vi "Set Project Path.vi"(10 "Top Level Path":path, 11 "Message Enqueuer in":refnum<class "Message Enqueuer.lvclass">) -> (3 "Message Enqueuer out":refnum<class "Message Enqueuer.lvclass">)   [LabVIEW 2013]
uses:
  <vilib>/ActorFramework/Message Enqueuer/Message Enqueuer.lvclass
  Models/Abstract Model Messages/Set Top Level Path Msg/Set Top Level Path Msg.lvclass/Set Top Level Path Msg.ctl
  <vilib>/ActorFramework/Message Enqueuer/Message Enqueuer.lvclass/Message Enqueuer.ctl
  <vilib>/ActorFramework/Message Enqueuer/Enqueue.vi
  <vilib>/ActorFramework/Message Priority Queue/Priority Enqueue.vi
  Models/Abstract Model Messages/Set Top Level Path Msg/Set Top Level Path Msg.lvclass
  <vilib>/ActorFrameworkMVC/UI Controller Messages/Get Model Actor Enqueuer Msg/Get Model Actor Enqueuer Msg.lvclass
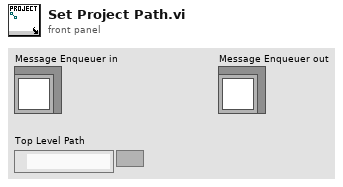
[diagram p1: front panel]
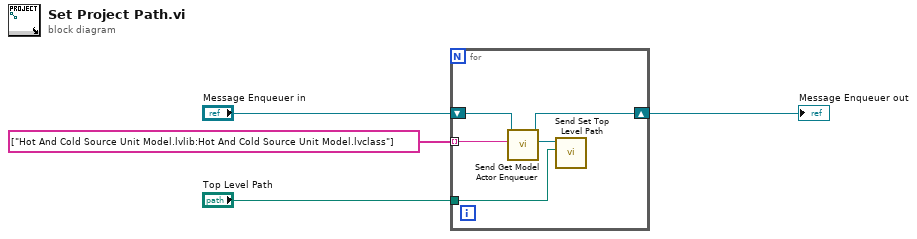
[diagram p0: block diagram]
diagram:
  n1 = for {
    tunnel: "Top Level Path" -> [w8]
    shift-right: [w6] -> w2
    shift-left: "Message Enqueuer in" -> [w7]
    tunnel: string[] ["Hot And Cold Source Unit Model.lvlib:Hot And Cold Source Unit Model.lvclass"] -> [w5] mode=indexing
    n2 = call <vilib>:"Send Get Model Actor Enqueuer.vi"("Model Name"=w5, "Message Enqueuer in"=w7) -> ("Reply"=w9:refnum<class "Message Enqueuer.lvclass">, "Message Enqueuer out"=w6:refnum<class "Message Enqueuer.lvclass">)  [unwired: 6 in, 2 out]
    n3 = call "Send Set Top Level Path.vi"("Top Level Path"=w8, "Message Enqueuer"=w9) -> ()  [unwired: 8 in, 2 out]
  }
  "Message Enqueuer out" <- w2
